vi "Send and Receive.vi"(6 "timeout (ms) [500]":i32, 8 "error in (no error)":errorcluster, 9 "params":variant, 10 "Command":string, 11 "Instrument in":refnum<class "Instrument.lvclass">) -> (0 "error out":errorcluster, 1 "Data out":variant, 2 "Command out":string, 3 "Instrument out":refnum<class "Instrument.lvclass">)   [LabVIEW 2019, in "Instrument.lvclass"]
uses:
  Instrument.lvclass
  Instrument.lvclass/Instrument.ctl
  RemoteControl/RemoteControl.lvclass
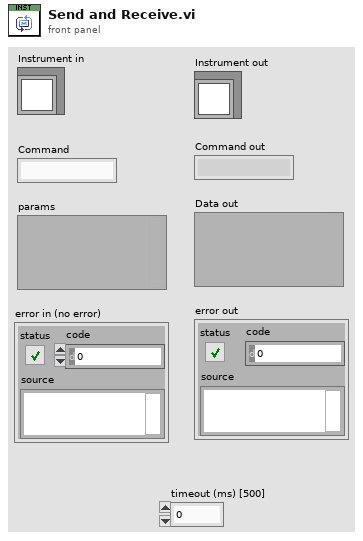
[diagram p1: front panel]
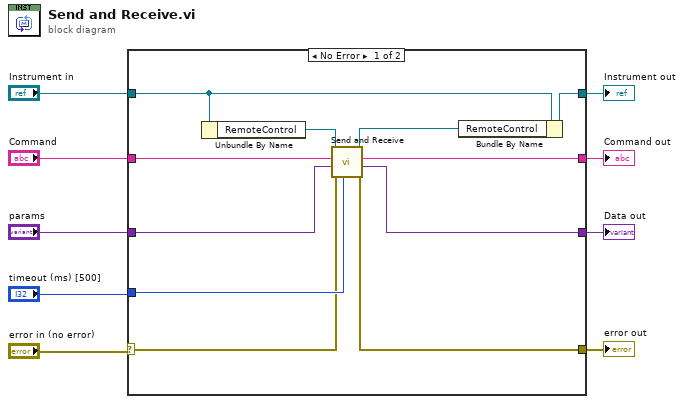
[diagram p0: block diagram]
diagram:
  n1 = case shown="No Error" "error in (no error)" {
    selector: "error in (no error)" -> [w10 w24]
    tunnel: "Instrument in" -> [w18 w23]
    tunnel: "timeout (ms) [500]" -> [w17 _]
    tunnel: "params" -> [w16 w21]
    tunnel: "Command" -> [w15 w22]
    tunnel: [w14 w23] -> w5
    tunnel: [w13 w24] -> w4
    tunnel: [w12 w22] -> w3
    tunnel: [w11 w21] -> w2
    frame No Error {
      n2 = Unbundle By Name(w18) -> ("RemoteControl"=w19:refnum<class "RemoteControl.lvclass">)
      n3 = call "Send and Receive.vi"("timeout (ms) [500]"=w17, "error in (no error)"=w10, "Data"=w16, "Command"=w15, "RemoteControl in"=w19) -> ("error out"=w13:errorcluster, "Data out"=w11:variant, "Command out"=w12:string, "RemoteControl out"=w20:refnum<class "RemoteControl.lvclass">)  [unwired: 3 in]
      n4 = Bundle By Name(cluster=w18, "RemoteControl"=w20) -> (w14:refnum<class "Instrument.lvclass">)
    }
    frame Error {
    }
  }
  "Data out" <- w2
  "error out" <- w4
  "Command out" <- w3
  "Instrument out" <- w5
